vi "NewCheesyDrive.vi"(4 "Track Width":dbl, 5 "Min Turn Radius":dbl, 6 "Tuning":dbl, 7 "Max Wheel Velocity":dbl, 10 "X":dbl(slide) scale=-1.0..1.0, 11 "Y":dbl(slide) scale=-1.0..1.0) -> (2 "Right Speed":dbl, 3 "Left Speed":dbl)   [LabVIEW 2018]
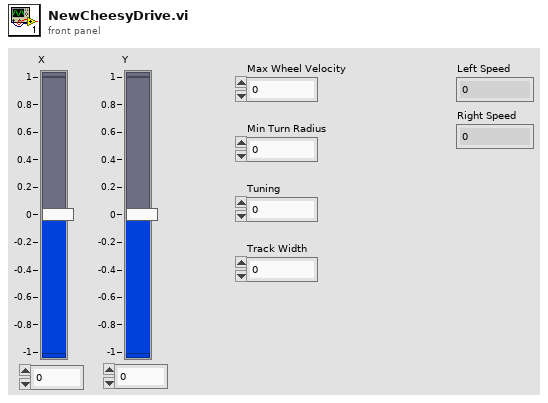
[diagram p1: front panel]
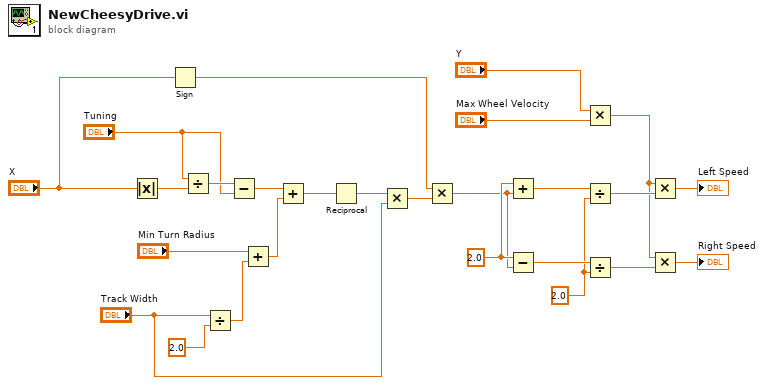
[diagram p0: block diagram]
diagram:
  w18 = 2.0 ("x")
  w21 = 2.0 ("x")
  n1 = Absolute Value(x="X") -> (abs(x)=w9:dbl)
  n2 = Sign(1:"X") -> (0:w1:dbl)
  n3 = Divide(x="Tuning", y=w9) -> (x/y=w25:dbl)
  n4 = Divide(x="Track Width", y=2.0 ("x")) -> (x/y=w7:dbl)
  n5 = Subtract(x=w25, y="Tuning") -> (x-y=w23:dbl)
  n6 = Add(x="Min Turn Radius", y=w7) -> (x+y=w10:dbl)
  n7 = Add(x=w23, y=w10) -> (x+y=w22:dbl)
  n8 = Reciprocal(x=w22) -> (1/x=w6:dbl)
  n9 = Multiply(x=w6, y="Track Width") -> (x*y=w3:dbl)
  n10 = Multiply(x=w1, y=w3) -> (x*y=w2:dbl)
  n11 = Add(x=w21, y=w2) -> (x+y=w20:dbl)
  n12 = Subtract(x=w21, y=w2) -> (x-y=w19:dbl)
  n13 = Multiply(x="Y", y="Max Wheel Velocity") -> (x*y=w15:dbl)
  n14 = Divide(x=w20, y=w18) -> (x/y=w17:dbl)
  n15 = Divide(x=w19, y=w18) -> (x/y=w16:dbl)
  n16 = Multiply(x=w15, y=w17) -> (x*y=→"Left Speed":dbl)
  n17 = Multiply(x=w15, y=w16) -> (x*y=→"Right Speed":dbl)
